vi "SCB Monitor-Controller - old shared var method.vi"() -> ()   [LabVIEW 2015]
uses:
  SC2 states.ctl
  Interface states.ctl
panel:
  in  "Tab Control":T1(tab)
  in  "Start Sample Change":bool
  out "Encoder Position":i32
  out "Converted Encoder":bool[](array[boolean])
  out "Raw Encoder":bool[](array[boolean])
  out "SC2 State Control":T2=enum."wait"
  in  "Requested Sample":u8
  in  "Encoder Offset":i16=-1021
  in  "error in (no error)":errorcluster
  out "error out":errorcluster
  in  "stop":bool
  in  "Random Change":bool
  out "Current Sample":u8
  out "Change Complete?":bool
  out "Monitor State":T3=enum."Wait"
  in  "Encoder Radius":dbl=2.0
  out "Encoder Radius Readback":dbl=2.0
  out "Encoder Destination":i32
  out "Motor status":bool=TRUE
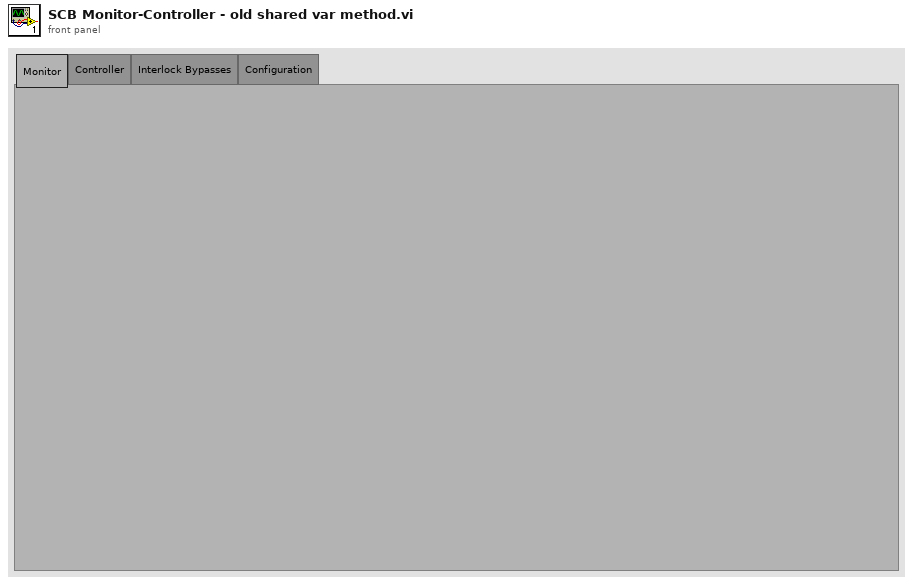
[diagram p1: front panel]
types:
  T1 = enum32{"Monitor", "Controller", "Interlock Bypasses", "Configuration"}
  T2 = typedef "SC2 states.ctl" = enum16{"initialize", "wait", "change sample start", "change sample", "check position", "rotate wheel", "sample change complete", "sample rod up", "sample rod down", "retract rod in", "retract rod out", "insert rod in", "insert rod out", "wheel GV open", "wheel GV close", "ion source GV open", "ion source GV close", "vent source", "pump source", "Shutdown"}
  T3 = typedef "Interface states.ctl" = enum16{"Initialization", "Wait", "start wheel change", "Shutdown"}
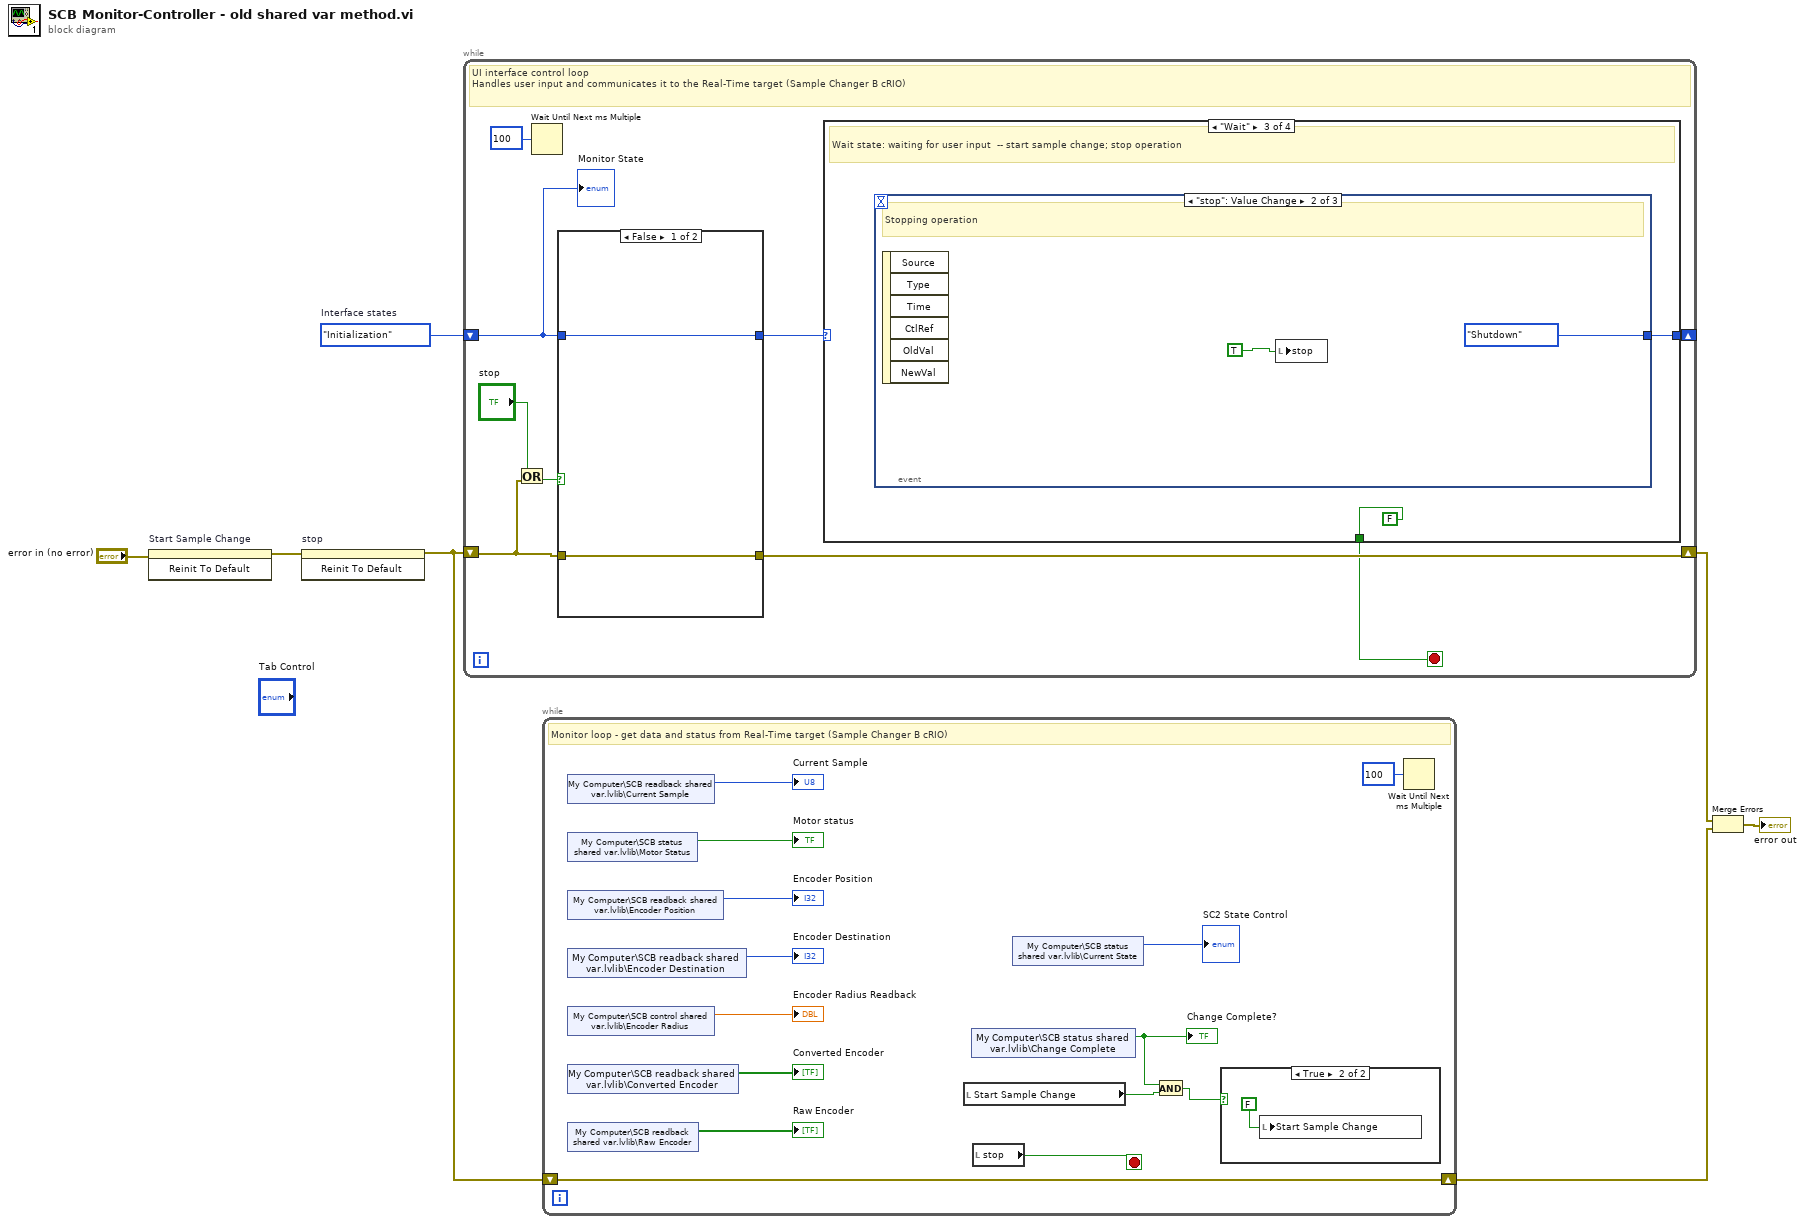
[diagram p0: block diagram]
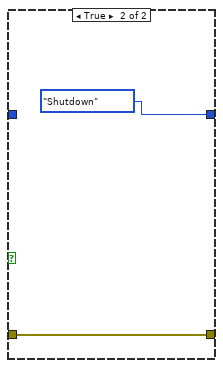
[diagram p3: hidden frame]
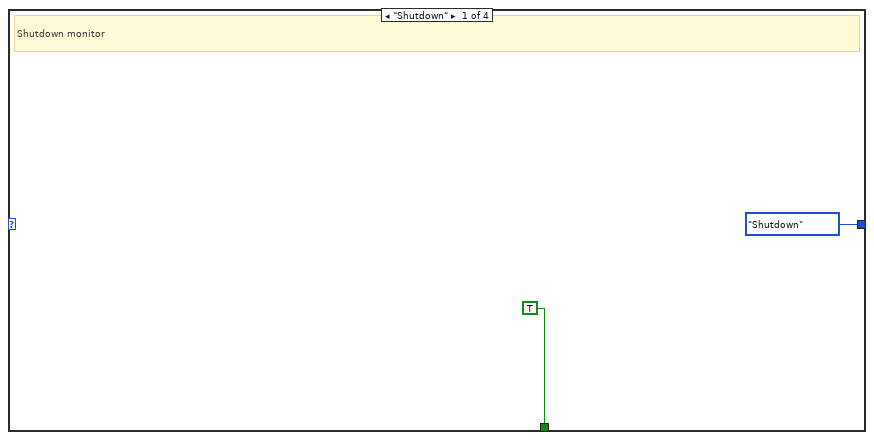
[diagram p4: hidden frame]
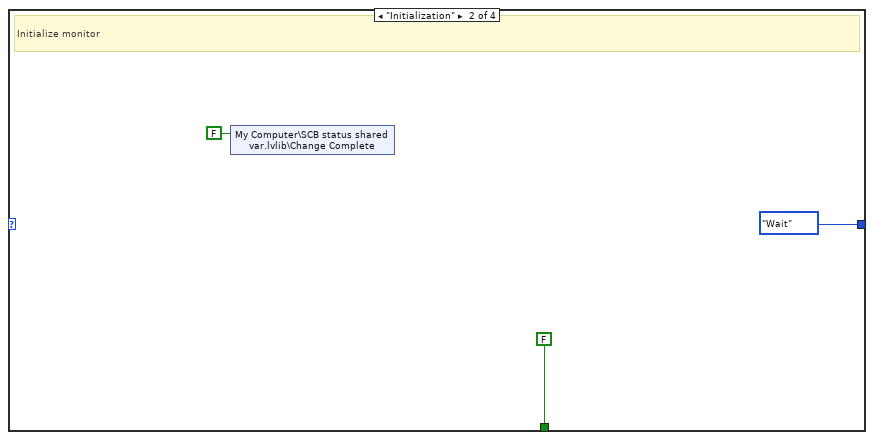
[diagram p5: hidden frame]
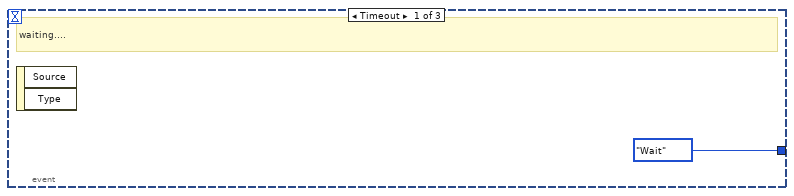
[diagram p6: hidden frame]
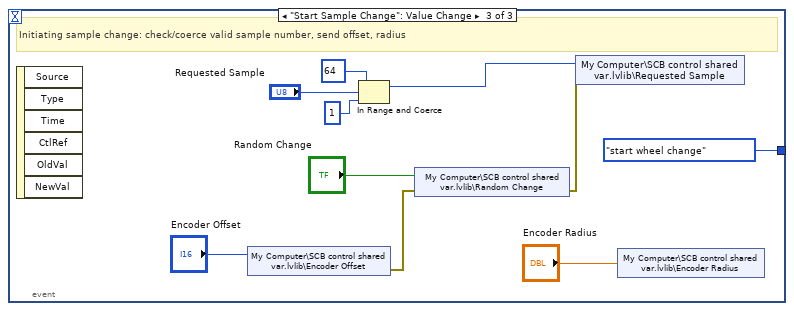
[diagram p7: hidden frame]
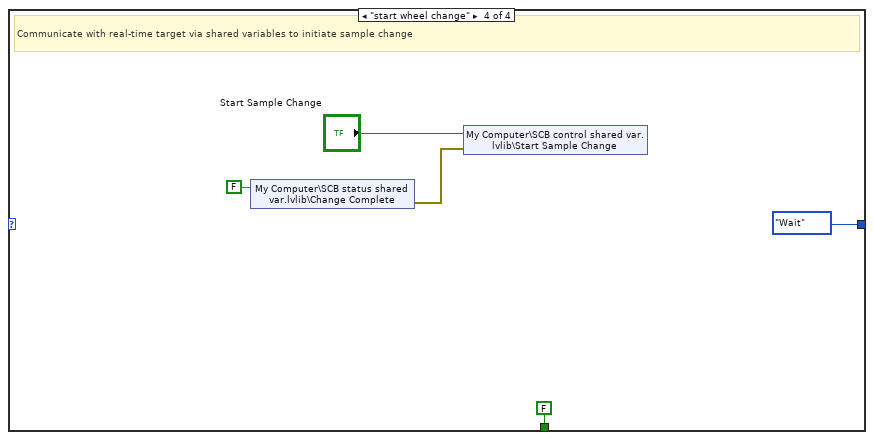
[diagram p8: hidden frame]
diagram:
  w4 = Interface_states."Initialization"  # Interface states
  n1 = invoke on="Start Sample Change" class="Bool (strict)" method="Reinit To Default"(error in="error in (no error)") -> (error out=w2:errorcluster)  [unwired: 2 in, 2 out]
  n2 = invoke on="stop" class="Bool (strict)" method="Reinit To Default"(error in=w2) -> (error out=w3:errorcluster)  [unwired: 2 in, 2 out]
  n3 = while {
    shift-right: [w13] -> w5
    shift-left: w3 -> [w9]
    shift-right: [w15] -> _
    shift-left: w4 -> [w11]
    stop <- w8 stop-if-true
    # "UI interface control loop\nHandles user input and communicates it to the Real-Time target (Sample Changer B cRIO)"
    n4 = Or(x="stop", y=w9) -> (x .or. y?=w10:bool)
    n5 = Wait Until Next ms Multiple(millisecond multiple=u32 100) -> ()  [unwired: 1 out]
    n6 = case shown="False" w10 {
      tunnel: w9 -> [w18 w19]
      tunnel: [w18 w19] -> w13
      tunnel: [w17 Interface_states."Shutdown" ("Interface states")] -> w12
      tunnel: w11 -> [w17 _]
      frame False {
      }
      frame True {
      }
    }
    n7 = case shown="\"Wait\"" w12 {
      tunnel: [Interface_states."Shutdown" ("Interface states") Interface_states."Wait" ("Interface states") w26 Interface_states."Wait" ("Interface states")] -> w15
      tunnel: [TRUE FALSE FALSE FALSE] -> w8
      frame "Shutdown" {
        # "Shutdown monitor"
      }
      frame "Initialization" {
        # "Initialize monitor"
        n8 = shared-variable "My Computer\\SCB status shared var.lvlib\\Change Complete"(FALSE ("SC2 Change Complete")) -> ()  [unwired: 1 in, 1 out]
      }
      frame "Wait" {
        # "Wait state: waiting for user input  -- start sample change; stop operation"
        n9 = event shown="[1] \"stop\": Value Change" {
          selector: _ -> [_ _ _]
          dyn-events: _ -> [_ _ _]
          timeout: _ -> [_ _ _]
          tunnel: [Interface_states."Wait" ("Interface states") Interface_states."Shutdown" ("Interface states") Interface_states."start wheel change" ("Interface states")] -> w26
          event Timeout {
            # "waiting...."
            n10 = event-data() -> ()  [unwired: 1 in, 2 out]
          }
          event "stop": Value Change {
            # "Stopping operation"
            n11 = event-data() -> ()  [unwired: 1 in, 6 out]
            n12 = local write "stop"(TRUE ("stop")) -> ()
          }
          event "Start Sample Change": Value Change {
            # "Initiating sample change: check/coerce valid sample number, send offset, radius"
            n13 = event-data() -> ()  [unwired: 1 in, 6 out]
            n14 = shared-variable "My Computer\\SCB control shared var.lvlib\\Encoder Offset"("Encoder Offset") -> (error out=w32:errorcluster)  [unwired: 1 in]
            n15 = In Range and Coerce(upper limit=u8 64, x="Requested Sample", lower limit=u8 1) -> (coerced(x)=w38:u8)  [unwired: 1 out]
            n16 = shared-variable "My Computer\\SCB control shared var.lvlib\\Random Change"("Random Change", error in=w32) -> (error out=w34:errorcluster)
            n17 = shared-variable "My Computer\\SCB control shared var.lvlib\\Requested Sample"(w38, error in=w34) -> ()  [unwired: 1 out]
            n18 = shared-variable "My Computer\\SCB control shared var.lvlib\\Encoder Radius"("Encoder Radius") -> ()  [unwired: 1 in, 1 out]
          }
        }
      }
      frame "start wheel change" {
        # "Communicate with real-time target via shared variables to initiate sample change"
        n19 = shared-variable "My Computer\\SCB status shared var.lvlib\\Change Complete"(FALSE ("SC2 Change Complete")) -> (error out=w41:errorcluster)  [unwired: 1 in]
        n20 = shared-variable "My Computer\\SCB control shared var.lvlib\\Start Sample Change"("Start Sample Change", error in=w41) -> ()  [unwired: 1 out]
      }
    }
    "Monitor State" <- w11
  }
  n21 = while {
    shift-right: [w58] -> w6
    shift-left: w3 -> [w58]
    stop <- w57 stop-if-true
    # "Monitor loop - get data and status from Real-Time target (Sample Changer B cRIO)"
    n22 = shared-variable "My Computer\\SCB readback shared var.lvlib\\Current Sample"() -> (→"Current Sample":u8)  [unwired: 1 in, 1 out]
    n23 = shared-variable "My Computer\\SCB status shared var.lvlib\\Motor Status"() -> (→"Motor status":bool)  [unwired: 1 in, 1 out]
    n24 = shared-variable "My Computer\\SCB readback shared var.lvlib\\Encoder Position"() -> (→"Encoder Position":i32)  [unwired: 1 in, 1 out]
    n25 = shared-variable "My Computer\\SCB readback shared var.lvlib\\Encoder Destination"() -> (→"Encoder Destination":i32)  [unwired: 1 in, 1 out]
    n26 = shared-variable "My Computer\\SCB control shared var.lvlib\\Encoder Radius"() -> (→"Encoder Radius Readback":dbl)  [unwired: 1 in, 1 out]
    n27 = shared-variable "My Computer\\SCB readback shared var.lvlib\\Converted Encoder"() -> (→"Converted Encoder":bool[])  [unwired: 1 in, 1 out]
    n28 = shared-variable "My Computer\\SCB readback shared var.lvlib\\Raw Encoder"() -> (→"Raw Encoder":bool[])  [unwired: 1 in, 1 out]
    n29 = local read "Start Sample Change"() -> (w55:bool)
    n30 = shared-variable "My Computer\\SCB status shared var.lvlib\\Change Complete"() -> (w51:bool)  [unwired: 1 in, 1 out]
    "Change Complete?" <- w51
    n31 = local read "stop"() -> (w57:bool)
    n32 = shared-variable "My Computer\\SCB status shared var.lvlib\\Current State"() -> (→"SC2 State Control":u16)  [unwired: 1 in, 1 out]
    n33 = And(x=w51, y=w55) -> (x .and. y?=w56:bool)
    n34 = case shown="True" w56 {
      frame False {
      }
      frame True {
        n35 = local write "Start Sample Change"(FALSE ("Start Sample Change")) -> ()
      }
    }
    n36 = Wait Until Next ms Multiple(millisecond multiple=u32 100) -> ()  [unwired: 1 out]
  }
  n37 = Merge Errors(w5, w6) -> (→"error out":errorcluster)
